vi "set configuration.vi"(8 "error in (no error)":errorcluster, 11 "DAQOrcaFlash in":refnum<class "DAQOrcaFlash.lvclass">) -> (0 "error out":errorcluster, 3 "DAQOrcaFlash out":refnum<class "DAQOrcaFlash.lvclass">)   [LabVIEW 2012, in "DAQOrcaFlash.lvclass"]
uses:
  DAQOrcaFlash.lvclass
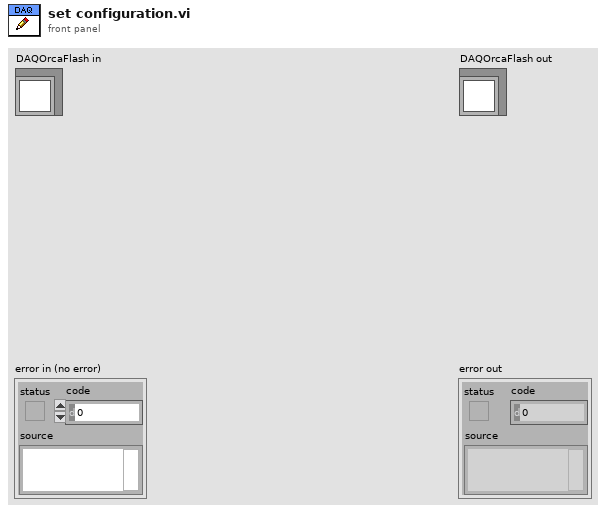
[diagram p1: front panel]
types:
  T1 = typedef "DAQOrcaFlash.lvclass/sensor_mode.ctl" = sgl
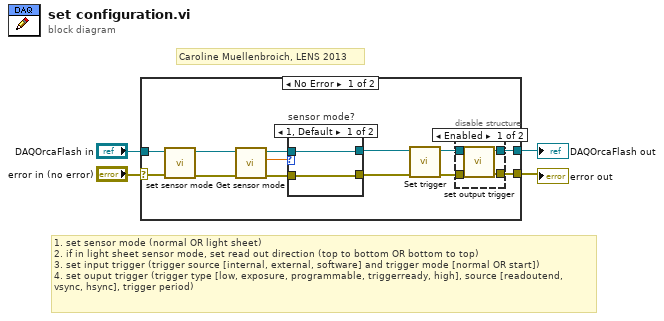
[diagram p0: block diagram]
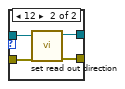
[diagram p3: hidden frame]
diagram:
  # "Caroline Muellenbroich, LENS 2013"
  # "1. set sensor mode (normal OR light sheet)\n2. if in light sheet sensor mode, set read out direction (top to bottom OR bottom to top)\n3. set input trigger (trigger source [internal, external, software] and trigger mode [normal OR start]) \n4. set ouput trigger (trigger type [low, exposure, programmable, triggerready, high], source [readoutend, vsync, hsync], trigger period)"
  n1 = case shown="No Error" "error in (no error)" {
    selector: "error in (no error)" -> [w17 w31]
    tunnel: [w12 w31] -> w1
    tunnel: [w13 w30] -> w2
    tunnel: "DAQOrcaFlash in" -> [w16 w30]
    frame No Error {
      n2 = call-dynamic "set sensor mode.vi"("error in (no error)"=w17, "DAQOrcaFlash in"=w16) -> ("error out"=w9:errorcluster, "DAQOrcaFlash out"=w7:refnum<class "DAQOrcaFlash.lvclass">)  [unwired: 8 in]
      n3 = call-dynamic "Get sensor mode.vi"("error in (no error)"=w9, "DAQOrcaFlash in"=w7) -> ("error out"=w8:errorcluster, "Sensor mode"=w5:T1, "DAQOrcaFlash out"=w6:refnum<class "DAQOrcaFlash.lvclass">)  [unwired: 7 in]
      n4 = case "sensor mode?" shown="1, Default" w5 {
        tunnel: w8 -> [w25 w29]
        tunnel: w6 -> [w24 w28]
        tunnel: [w24 w27] -> w11
        tunnel: [w25 w26] -> w10
        frame 1, Default {
        }
        frame 12 {
          n5 = call-dynamic "set read out direction.vi"("error in (no error)"=w29, "DAQOrcaFlash in"=w28) -> ("error out"=w26:errorcluster, "DAQOrcaFlash out"=w27:refnum<class "DAQOrcaFlash.lvclass">)  [unwired: 8 in]
        }
      }
      n6 = call-dynamic "Set trigger.vi"("error in (no error)"=w10, "DAQOrcaFlash in"=w11) -> ("error out"=w14:errorcluster, "DAQOrcaFlash out"=w15:refnum<class "DAQOrcaFlash.lvclass">)  [unwired: 8 in]
      n7 = disable-structure shown="Enabled" {
        disable-tunnel: w15 -> [w21 w22]
        disable-tunnel: w14 -> [w20 w23]
        disable-tunnel: [w19 w22] -> w13
        disable-tunnel: [w18 w23] -> w12
        frame Enabled {
          n8 = call-dynamic "set output trigger.vi"("error in (no error)"=w20, "DAQOrcaFlash in"=w21) -> ("error out"=w18:errorcluster, "DAQOrcaFlash out"=w19:refnum<class "DAQOrcaFlash.lvclass">)  [unwired: 8 in]
        }
        frame Disabled {
        }
      }
    }
    frame Error {
    }
  }
  "error out" <- w1
  "DAQOrcaFlash out" <- w2
